vi "DefaultClientDataFolder.vi"(8 "error in (no error)":errorcluster, 11 "TCP_Client in":refnum<class "TCP_Client.lvclass">) -> (0 "error out":errorcluster, 3 "TCP_Client out":refnum<class "TCP_Client.lvclass">)   [LabVIEW 2023, in "TCP_Client.lvlib" / "TCP_Client.lvclass"]
uses:
  TCP_Client.lvclass
  <vilib>/Utility/sysdir.llb/System Directory Type.ctl
  TCP_Client.lvclass/TCP_Client.ctl
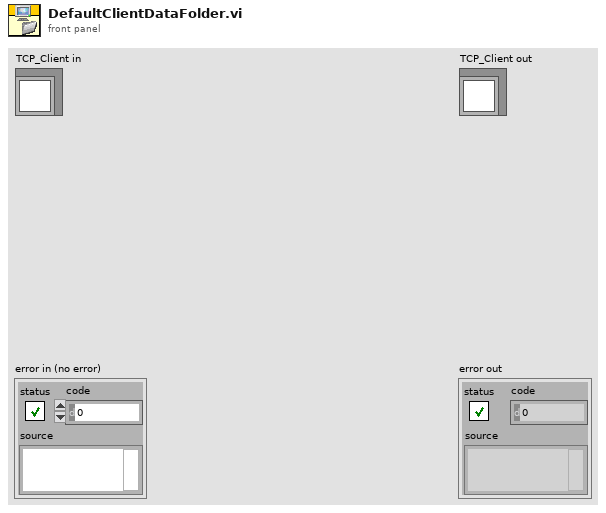
[diagram p1: front panel]
types:
  T1 = typedef "System Directory Type.ctl" = i32
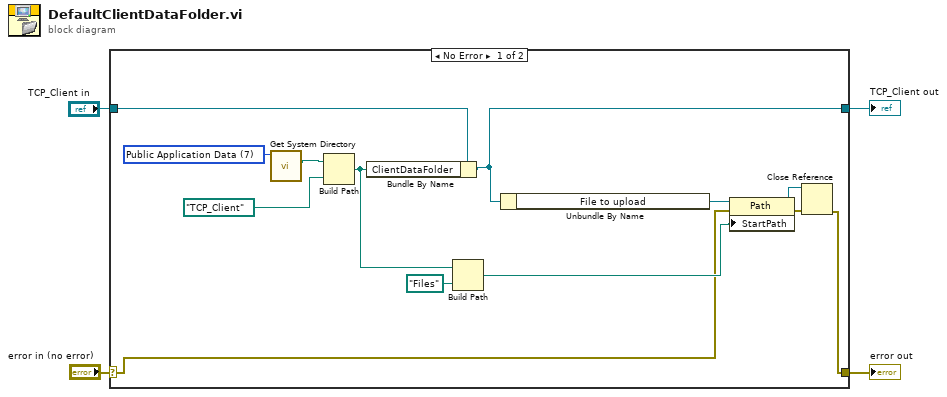
[diagram p0: block diagram]
diagram:
  n1 = case shown="No Error" "error in (no error)" {
    selector: "error in (no error)" -> [w8 w19]
    tunnel: [w5 w19] -> w3
    tunnel: [w13 w18] -> w1
    tunnel: "TCP_Client in" -> [w14 w18]
    frame No Error {
      w17 = T1 7 items=["User Home"=0, "User Desktop"=1, "User Documents"=2, "User Application Data"=3, "User Preferences"=4, "User Temporary"=5, "Public Documents"=6, "Public Application Data"=7, "Public Preferences"=8, "Public Cache"=13, "System Core Libraries"=9, "System Installed Libraries"=10, "Application Files"=11, "Boot Volume Root"=12] ("system directory type")
      n2 = call <vilib>:"Get System Directory.vi"("system directory type"=w17) -> ("system directory"=w16:path)  [unwired: 10 in]
      n3 = Build Path(base path=w16, name or relative path=path "TCP_Client") -> (appended path=w11:path)
      n4 = Bundle By Name(cluster=w14, "ClientDataFolder"=w11) -> (w13:refnum<class "TCP_Client.lvclass">)
      n5 = Build Path(base path=w11, name or relative path=path "Files") -> (appended path=w9:path)
      n6 = Unbundle By Name(w13) -> ("File to upload"=w12:refnum<vi>)
      n7 = property class="Path"(reference=w12, error in=w8, "StartPath"=w9) -> (reference out=w6:refnum<vi>, error out=w7:errorcluster)
      n8 = Close Reference(reference=w6, error in (no error)=w7) -> (error out=w5:errorcluster)
    }
    frame Error {
    }
  }
  "error out" <- w3
  "TCP_Client out" <- w1
